vi "Begin.vi"() -> (0 "error out":errorcluster)   [LabVIEW 2013]
doc: "Called before other user functions, this VI is expected to open initial I/O refnums, load in file data, and do all program initialization. Notice that the <B>error out</B> terminal is simply used for data flow. Wiring it to other structures or subVIs ensures that this VI runs first."
uses:
  <vilib>/Rock Robotics/WPI/DriverStation/WPI_DriverStationRobotMode2.ctl
  <vilib>/Rock Robotics/WPI/CAN/Jaguar/SubVIs/WPI_CANJaguar_ControlMode.ctl
  <vilib>/Rock Robotics/SystemInterfaces/CounterEncoderSourceConvertion/FPGA_CounterEncoderSourceConvertionLVSourceType.ctl
  <vilib>/Rock Robotics/SystemInterfaces/Typedef/FPGA_TypedefDigitalModule.ctl
  <vilib>/Rock Robotics/SystemInterfaces/DIO/FPGA_DIODigitalSourceChannel.ctl
  <vilib>/Rock Robotics/SystemInterfaces/AnalogTrigger/FPGA_AnalogTriggerIndex.ctl
  <vilib>/Rock Robotics/SystemInterfaces/AnalogTrigger/FPGA_AnalogTriggerOutType.ctl
  <vilib>/Rock Robotics/SystemInterfaces/DIO/FPGA_DIOPWMChannel.ctl
  <vilib>/Rock Robotics/WPI/SafetyOutput/WPI_SafetyOutputConfigMenu.ctl
  Robot Global Data.vi
  <vilib>/Rock Robotics/WPI/MotorControl/WPI_MotorControlOpenCANJaguar.vi
  <vilib>/Rock Robotics/WPI/RobotDrive/WPI_RobotDriveOpen4MotorWithExistingMotors.vi
  <vilib>/Rock Robotics/WPI/MotorControl/WPI_MotorControlOpen Victor.vi
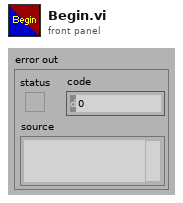
[diagram p1: front panel]
types:
  T1 = typedef "WPI_SafetyOutputConfigMenu.ctl" = enum16{"Enable", "Disable"}
  T2 = typedef "FPGA_DIOPWMChannel.ctl" = enum8{"PWM 1", "PWM 2", "PWM 3", "PWM 4", "PWM 5", "PWM 6", "PWM 7", "PWM 8", "PWM 9", "PWM 10", "Invalid"}
  T3 = typedef "FPGA_CounterEncoderSourceConvertionLVSourceType.ctl" = cluster{"DevStatus":errorcluster, "AnalogTriggerMode?":bool, "DigitalMode":cluster{"Digital Module":T4, "DIO Channel":T5}, "AnalogTriggerMode":cluster{"AnalogTriggerIndex":T6, "OutputType":T7}}
  T4 = typedef "FPGA_TypedefDigitalModule.ctl" = enum16{"Digital Module 1", "Digital Module 2"}
  T5 = typedef "FPGA_DIODigitalSourceChannel.ctl" = enum8{"DIO 1", "DIO 2", "DIO 3", "DIO 4", "DIO 5", "DIO 6", "DIO 7", "DIO 8", "DIO 9", "DIO 10", "DIO 11", "DIO 12", "DIO 13", "DIO 14", "Disabled"}
  T6 = typedef "FPGA_AnalogTriggerIndex.ctl" = enum8{"Trig 0", "Trig 1", "Trig 2", "Trig 3", "Trig 4", "Trig 5", "Trig 6", "Trig 7", "Invalid"}
  T7 = typedef "FPGA_AnalogTriggerOutType.ctl" = enum16{"InWindow", "TriggerState", "Rising", "Falling"}
  T8 = typedef "WPI_CANJaguar_ControlMode.ctl" = enum8{"Percent VBus", "Current", "Speed", "Position", "Voltage"}
  T9 = typedef "WPI_DriverStationRobotMode2.ctl" = enum16{"Autonomous Disabled", "Autonomous Enabled", "Teleop Disabled", "Teleop Enabled", "Timeout", "Finish", "Test Disabled", "Test Enabled"}
  T10 = typedef "WPI_MotorControlDeviceRef.ctl" = cluster{"DeviceStatus":errorcluster, "Type":enum16{"PWM", "CAN"}, "PWM":cluster{"Digital Module":T4, "PWM Channel":T2, "DeadBand":T11}, "CAN":cluster{"Device Number":u8, "Control Mode":T8, "Semaphore":T12, "Max Vout":dbl}, "Invert":bool, "TransformRef":T13, "InvTransformRef":T13}
  T11 = typedef "WPI_PWMDeadband.ctl" = cluster{"Name":string, "maxPositivePwm":i32, "minPositivePwm":i32, "centerPwm":i32, "maxNegativePwm":i32, "minNegativePwm":i32, "angularRange":u16}
  T12 = typedef "Semaphore RefNum" = refnum<k1>
  T13 = typedef "WPI_PWMTransform_ConPane.ctl" = refnum<vi>
  T14 = typedef "WPI_EncoderDevRef.ctl" = cluster{"DevStatus":errorcluster, "EncoderIndex":T15, "CounterIndex":T16, "DistancePerCount":dbl, "Decoding Type":T17}
  T15 = typedef "FPGA_EncoderIdx.ctl" = enum8{"Enc 0", "Enc 1", "Enc 2", "Enc 3", "Invalid"}
  T16 = typedef "FPGA_CounterCtrSystemIndex.ctl" = enum8{"Ctr 0", "Ctr 1", "Ctr 2", "Ctr 3", "Ctr 4", "Ctr 5", "Ctr 6", "Ctr 7", "Invalid"}
  T17 = typedef "WPI_EncoderType.ctl" = enum16{"1x", "2x", "4x"}
  T18 = typedef "WPI_RobotDriveDevRef.ctl" = cluster{"DevStatus":errorcluster, "Motors[]":T10[], "Square Inputs":bool, "Max Output":dbl, "Isochronous":bool}
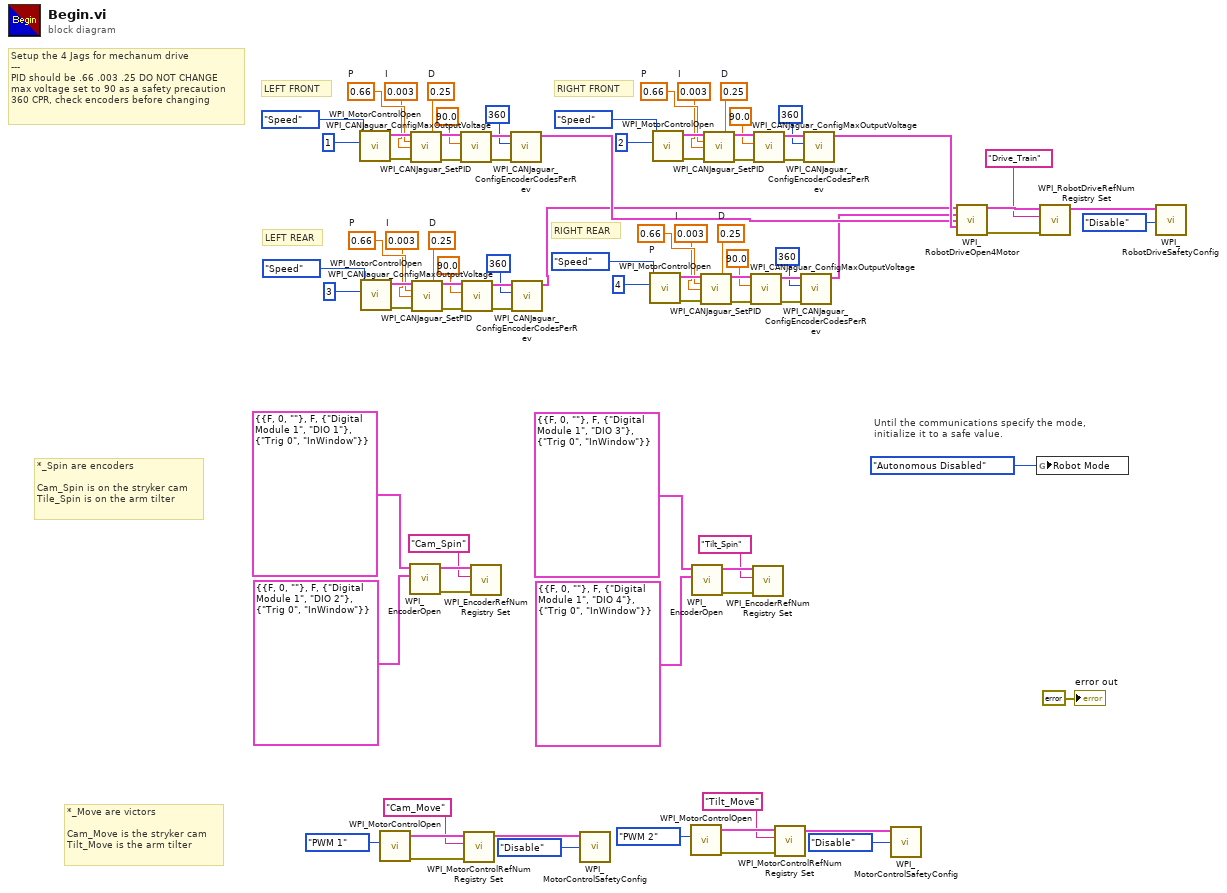
[diagram p0: block diagram]
diagram:
  w27 = 0.25  # D
  w28 = 0.003  # I
  w29 = 0.66  # P
  w40 = 0.25  # D
  w41 = 0.003  # I
  w42 = 0.66  # P
  w53 = 0.25  # D
  w54 = 0.003  # I
  w55 = 0.66  # P
  w66 = 0.25  # D
  w67 = 0.003  # I
  w68 = 0.66  # P
  # "*_Move are victors\n\nCam_Move is the stryker cam\nTilt_Move is the arm tilter"
  # "*_Spin are encoders\n\nCam_Spin is on the stryker cam\nTile_Spin is on the arm tilter"
  # "LEFT REAR"
  # "RIGHT REAR"
  # "RIGHT FRONT"
  # "LEFT FRONT"
  # "Until the communications specify the mode,\ninitialize it to a safe value."
  # "Setup the 4 Jags for mechanum drive\n---\nPID should be .66 .003 .25 DO NOT CHANGE\nmax voltage set to 90 as a safety precaution\n360 CPR, check encoders before changing"
  n1 = call-poly <vilib>:"WPI_MotorControlOpen.vi"("Device Number"=u8 1, "Control Mode"=WPI_CANJaguar_ControlMode."Speed") -> ("error out"=w75:errorcluster, "MotorControlDeviceRef"=w76:T10)  [unwired: 8 in]
  n2 = call-poly <vilib>:"WPI_MotorControlOpen.vi"("Device Number"=u8 3, "Control Mode"=WPI_CANJaguar_ControlMode."Speed") -> ("error out"=w36:errorcluster, "MotorControlDeviceRef"=w37:T10)  [unwired: 8 in]
  n3 = call-poly <vilib>:"WPI_MotorControlOpen.vi"("PWM Channel"=FPGA_DIOPWMChannel."PWM 1") -> ("error out"=w10:errorcluster, "MotorControlDeviceRef"=w11:T10)  [unwired: 9 in]
  n4 = call <vilib>:"WPI_EncoderOpen.vi"("BSource"=T3 {"DevStatus"={"status"=FALSE, "code"=0, "source"=""}, "AnalogTriggerMode?"=FALSE, "DigitalMode"={"Digital Module"=enum."Digital Module 1", "DIO Channel"=enum."DIO 2"}, "AnalogTriggerMode"={"AnalogTriggerIndex"=enum."Trig 0", "OutputType"=enum."InWindow"}}, "ASource"=T3 {"DevStatus"={"status"=FALSE, "code"=0, "source"=""}, "AnalogTriggerMode?"=FALSE, "DigitalMode"={"Digital Module"=enum."Digital Module 1", "DIO Channel"=enum."DIO 1"}, "AnalogTriggerMode"={"AnalogTriggerIndex"=enum."Trig 0", "OutputType"=enum."InWindow"}}) -> ("error out"=w20:errorcluster, "EncoderDevRef"=w19:T14)  [unwired: 8 in]
  n5 = call <vilib>:"WPI_CANJaguar_SetPID.vi"("CAN Jaguar Ref"=w76, "P"=w68, "I"=w67, "D"=w66, "error in (no error)"=w75) -> ("CAN Jaguar Ref Out"=w73:T10, "error out"=w74:errorcluster)  [unwired: 9 in]
  n6 = call <vilib>:"WPI_CANJaguar_SetPID.vi"("CAN Jaguar Ref"=w37, "P"=w29, "I"=w28, "D"=w27, "error in (no error)"=w36) -> ("CAN Jaguar Ref Out"=w34:T10, "error out"=w35:errorcluster)  [unwired: 9 in]
  n7 = call <vilib>:"WPI_CANJaguar_ConfigMaxOutputVoltage.vi"("error in (no error)"=w74, "Maximum Output Voltage"=90.0, "CAN Jaguar Ref"=w73) -> ("error out"=w72:errorcluster, "CAN Jaguar Ref Out"=w71:T10)  [unwired: 7 in]
  n8 = call <vilib>:"WPI_CANJaguar_ConfigMaxOutputVoltage.vi"("error in (no error)"=w35, "Maximum Output Voltage"=90.0, "CAN Jaguar Ref"=w34) -> ("error out"=w33:errorcluster, "CAN Jaguar Ref Out"=w32:T10)  [unwired: 7 in]
  n9 = call <vilib>:"WPI_MotorControlRefNum Registry Set.vi"("error in (no error)"=w10, "refnum name"="Cam_Move", "MotorControlDevRef"=w11) -> ("MotorControlDevRef"=w1:T10)  [unwired: 7 in, 1 out]
  n10 = call <vilib>:"WPI_EncoderRefNum Registry Set.vi"("error in (no error)"=w20, "refnum name"="Cam_Spin", "EncoderDevRef"=w19) -> ()  [unwired: 7 in, 2 out]
  n11 = call <vilib>:"WPI_CANJaguar_ConfigEncoderCodesPerRev.vi"("error in (no error)"=w72, "Encoder Codes Per Rev"=u16 360, "CAN Jaguar Ref"=w71) -> ("CAN Jaguar Ref Out"=w25:T10)  [unwired: 7 in, 1 out]
  n12 = call <vilib>:"WPI_CANJaguar_ConfigEncoderCodesPerRev.vi"("error in (no error)"=w33, "Encoder Codes Per Rev"=u16 360, "CAN Jaguar Ref"=w32) -> ("CAN Jaguar Ref Out"=w24:T10)  [unwired: 7 in, 1 out]
  n13 = call <vilib>:"WPI_MotorControlSafetyConfig.vi"("mode"=WPI_SafetyOutputConfigMenu."Disable", "MotorControlDevRef"=w1) -> ()  [unwired: 8 in, 2 out]
  n14 = call-poly <vilib>:"WPI_MotorControlOpen.vi"("Device Number"=u8 4, "Control Mode"=WPI_CANJaguar_ControlMode."Speed") -> ("error out"=w49:errorcluster, "MotorControlDeviceRef"=w50:T10)  [unwired: 8 in]
  n15 = call-poly <vilib>:"WPI_MotorControlOpen.vi"("Device Number"=u8 2, "Control Mode"=WPI_CANJaguar_ControlMode."Speed") -> ("error out"=w62:errorcluster, "MotorControlDeviceRef"=w63:T10)  [unwired: 8 in]
  n16 = call-poly <vilib>:"WPI_MotorControlOpen.vi"("PWM Channel"=FPGA_DIOPWMChannel."PWM 2") -> ("error out"=w6:errorcluster, "MotorControlDeviceRef"=w7:T10)  [unwired: 9 in]
  n17 = call <vilib>:"WPI_EncoderOpen.vi"("BSource"=T3 {"DevStatus"={"status"=FALSE, "code"=0, "source"=""}, "AnalogTriggerMode?"=FALSE, "DigitalMode"={"Digital Module"=enum."Digital Module 1", "DIO Channel"=enum."DIO 4"}, "AnalogTriggerMode"={"AnalogTriggerIndex"=enum."Trig 0", "OutputType"=enum."InWindow"}}, "ASource"=T3 {"DevStatus"={"status"=FALSE, "code"=0, "source"=""}, "AnalogTriggerMode?"=FALSE, "DigitalMode"={"Digital Module"=enum."Digital Module 1", "DIO Channel"=enum."DIO 3"}, "AnalogTriggerMode"={"AnalogTriggerIndex"=enum."Trig 0", "OutputType"=enum."InWindow"}}) -> ("error out"=w15:errorcluster, "EncoderDevRef"=w14:T14)  [unwired: 8 in]
  n18 = call <vilib>:"WPI_CANJaguar_SetPID.vi"("CAN Jaguar Ref"=w50, "P"=w42, "I"=w41, "D"=w40, "error in (no error)"=w49) -> ("CAN Jaguar Ref Out"=w47:T10, "error out"=w48:errorcluster)  [unwired: 9 in]
  n19 = call <vilib>:"WPI_CANJaguar_SetPID.vi"("CAN Jaguar Ref"=w63, "P"=w55, "I"=w54, "D"=w53, "error in (no error)"=w62) -> ("CAN Jaguar Ref Out"=w60:T10, "error out"=w61:errorcluster)  [unwired: 9 in]
  n20 = call <vilib>:"WPI_CANJaguar_ConfigMaxOutputVoltage.vi"("error in (no error)"=w48, "Maximum Output Voltage"=90.0, "CAN Jaguar Ref"=w47) -> ("error out"=w46:errorcluster, "CAN Jaguar Ref Out"=w45:T10)  [unwired: 7 in]
  n21 = call <vilib>:"WPI_EncoderRefNum Registry Set.vi"("error in (no error)"=w15, "refnum name"="Tilt_Spin", "EncoderDevRef"=w14) -> ()  [unwired: 7 in, 2 out]
  n22 = call <vilib>:"WPI_CANJaguar_ConfigMaxOutputVoltage.vi"("error in (no error)"=w61, "Maximum Output Voltage"=90.0, "CAN Jaguar Ref"=w60) -> ("error out"=w59:errorcluster, "CAN Jaguar Ref Out"=w58:T10)  [unwired: 7 in]
  n23 = call <vilib>:"WPI_MotorControlRefNum Registry Set.vi"("error in (no error)"=w6, "refnum name"="Tilt_Move", "MotorControlDevRef"=w7) -> ("MotorControlDevRef"=w4:T10)  [unwired: 7 in, 1 out]
  n24 = call <vilib>:"WPI_CANJaguar_ConfigEncoderCodesPerRev.vi"("error in (no error)"=w46, "Encoder Codes Per Rev"=u16 360, "CAN Jaguar Ref"=w45) -> ("CAN Jaguar Ref Out"=w23:T10)  [unwired: 7 in, 1 out]
  n25 = call <vilib>:"WPI_CANJaguar_ConfigEncoderCodesPerRev.vi"("error in (no error)"=w59, "Encoder Codes Per Rev"=u16 360, "CAN Jaguar Ref"=w58) -> ("CAN Jaguar Ref Out"=w26:T10)  [unwired: 7 in, 1 out]
  n26 = call <vilib>:"WPI_MotorControlSafetyConfig.vi"("mode"=WPI_SafetyOutputConfigMenu."Disable", "MotorControlDevRef"=w4) -> ()  [unwired: 8 in, 2 out]
  n27 = call-poly <vilib>:"WPI_RobotDriveOpen4Motor.vi"("Rear Left Motor Dev Ref"=w24, "Rear Right Motor Dev Ref"=w23, "Front Left Motor Dev Ref"=w25, "Front Right Motor Dev Ref"=w26) -> ("RobotDriveDevRef"=w85:T18, "error out"=w83:errorcluster)  [unwired: 10 in]
  n28 = global write "Robot Global Data.vi" "Robot Mode"(WPI_DriverStationRobotMode2."Autonomous Disabled" ("Robot Mode")) -> ()
  n29 = call <vilib>:"WPI_RobotDriveRefNum Registry Set.vi"("error in (no error)"=w83, "refnum name"="Drive_Train", "RobotDriveDevRef"=w85) -> ("RobotDriveDevRef"=w82:T18)  [unwired: 8 out]
  n30 = call <vilib>:"WPI_RobotDriveSafetyConfig.vi"("mode"=WPI_SafetyOutputConfigMenu."Disable", "RobotDriveDevRef"=w82) -> ()  [unwired: 8 in, 2 out]
  "error out" <- errorcluster {"status"=FALSE, "code"=0, "source"=""} ("error out")
